vi "File_Reader.vi"(7 "File Name With Extension":string, 9 "Path":path) -> (0 "error out":errorcluster, 1 "concatenated string":string, 2 "lowercase file extension":string, 3 "File Contents":string, 4 "file or folder exists?":bool, 5 "File status":string)   [LabVIEW 2012]
uses:
  <vilib>/Rock Robotics/WPI/DriverStation/DriverStationLCD/WPI_DriverStationLCDLCDLine.ctl
panel:
  # "Load file"
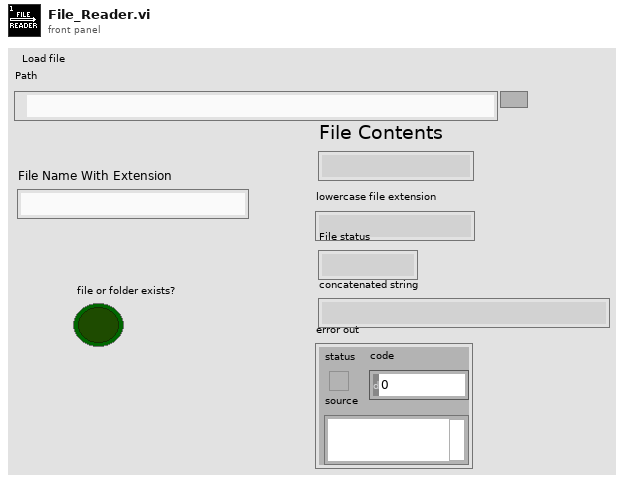
[diagram p1: front panel]
types:
  T1 = typedef "WPI_DriverStationLCDLCDLine.ctl" = enum16{"Main - Line 1", "User - Line 2", "User - Line 3", "User - Line 4", "User - Line 5", "User - Line 6"}
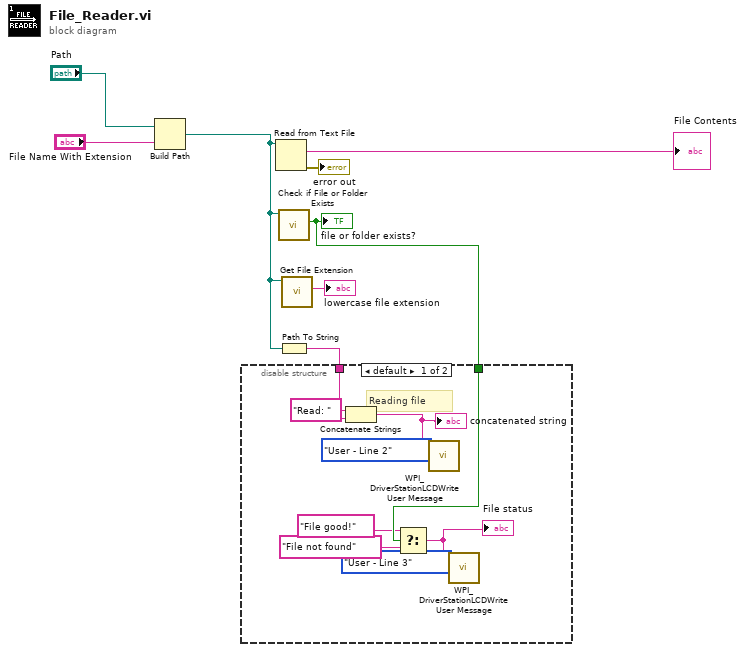
[diagram p0: block diagram]
diagram:
  n1 = Build Path(base path="Path", name or relative path="File Name With Extension") -> (appended path=w3:path)
  n2 = Read from Text File(file (use dialog)=w3) -> (text=→"File Contents":string, error out=→"error out":errorcluster)  [unwired: 2 in, 3 out]
  n3 = call <vilib>:"Check if File or Folder Exists.vi"("path"=w3) -> ("file or folder exists?"=w1:bool)  [unwired: 1 in, 9 out]
  "file or folder exists?" <- w1
  n4 = Path To String(path=w3) -> (string=w2:string)
  n5 = disable-structure shown="default" {
    disable-tunnel: w1 -> [w15 _]
    disable-tunnel: w2 -> [w10 _]
    frame condition #0 (active) {
      # "Reading file"
      n6 = Concatenate Strings("Read: " ("string"), w10) -> (w9:string)
      "concatenated string" <- w9
      n7 = Select(t="File good!", s=w15, f="File not found") -> (s? t:f=w13:string)
      "File status" <- w13
      n8 = call <vilib>:"WPI_DriverStationLCDWrite User Message.vi"("line text"=w9, "line"=WPI_DriverStationLCDLCDLine."User - Line 2") -> ()  [unwired: 3 in, 11 out]
      n9 = call <vilib>:"WPI_DriverStationLCDWrite User Message.vi"("line text"=w13, "line"=WPI_DriverStationLCDLCDLine."User - Line 3") -> ()  [unwired: 3 in, 11 out]
    }
    frame condition #1 {
    }
  }
  n10 = call <vilib>:"Get File Extension.vi"("file"=w3) -> ("lowercase file extension"=→"lowercase file extension":string)  [unwired: 1 in, 9 out]
